vi "DCAM_show_preview_update_camera.vi"() -> ()   [LabVIEW 2015]
panel:
  out "S Horiz Width":i32
  in  "Horizontal Width":i32 min=4 max=2048 step=4
  out "Image Preview":u16[][](graph) caption="Image"
  out "S Start Trig Mode":dbl
  out "S Binning":dbl
  in  "Start Trigger Mode":u32(ring)=1 items=["Internal"=1, "External Edge"=2, "External Level"=4, "Software"=32, "Fast Repetition"=64, "TDI"=128, "Trigger Start"=512, "Sync Readout"=1024]
  in  "Binning":u16(ring) items=["1x1"=1, "2x2"=2, "4x4"=4]
  out "S Vert Offset":i32
  out "S Horiz Offset":i32
  in  "Vertical Offset":i32 min=0 max=0 step=4
  in  "Horizontal Offset":i32 min=0 max=0 step=4
  in  "Scan Mode":dbl min=1.0 max=2.0 step=1.0
  out "S Scan Mode":dbl min=1.0 max=2.0 step=1.0
  in  "Exposure":dbl min=0.0010036691729323308 max=10.000004210526315 step=1e-08
  out "S Exposure":dbl
  out "S Vert Width":i32
  in  "Vertical Width":i32 min=4 max=2048 step=4
  out "error out":errorcluster
  out "DCAM Ver.":string
  out "Library Ver.":string
  out "Firmware":string
  out "Camera ID":string
  out "Model":string
  out "Timeseries Base Filename":string
  out "Timeseries Save Path":path
  in  "Start Button":bool
  out "Image":u16[][](graph)
  in  "Stop":bool
  out "Frames Recorded":i32
  in  "Frames":i32=100
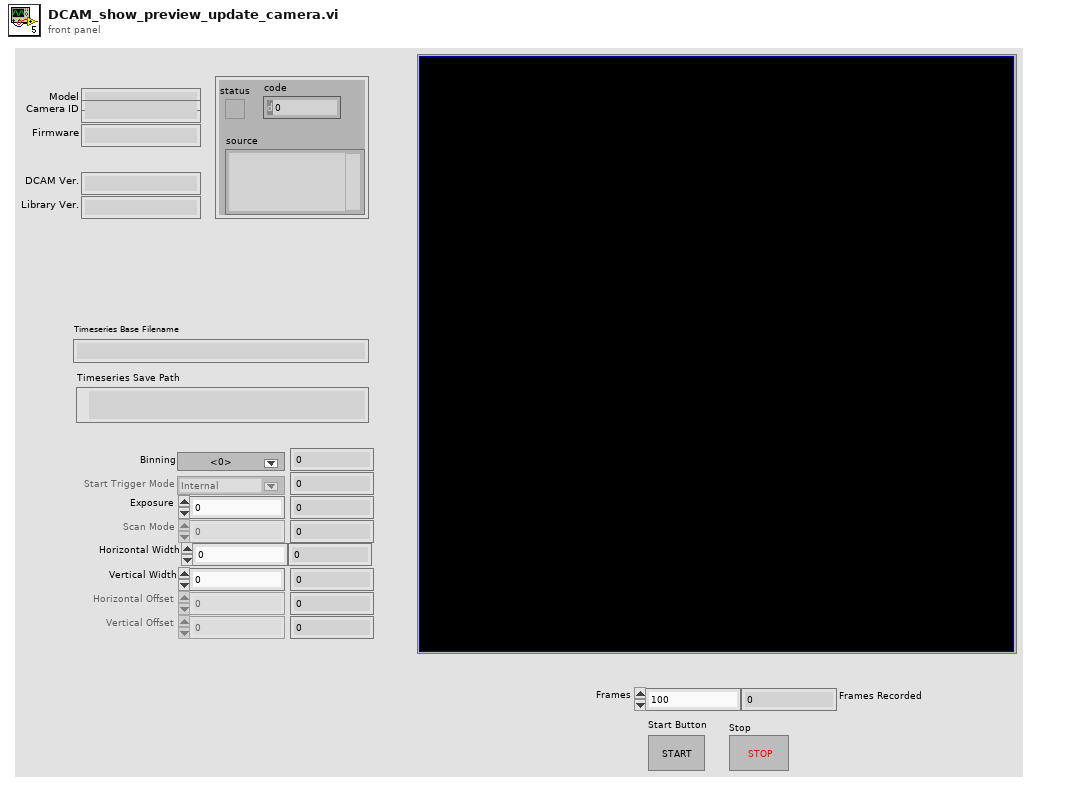
[diagram p1: front panel]
types:
  T1 = cluster{"Capture Library":string, "DCAM-API":string}
  T2 = cluster{"Model":string, "Camera ID":string, "Firmware":string}
  T3 = cluster{"Value":i32, "Minimum":i32, "Maximum":i32, "Increment":i32}
  T4 = cluster{"height":u32, "width":u32, "datatype":u32}
  T5 = cluster{"Horizontal Offset":i32, "Vertical Offset":i32, "Horizontal Width":i32, "Vertical Width":i32}
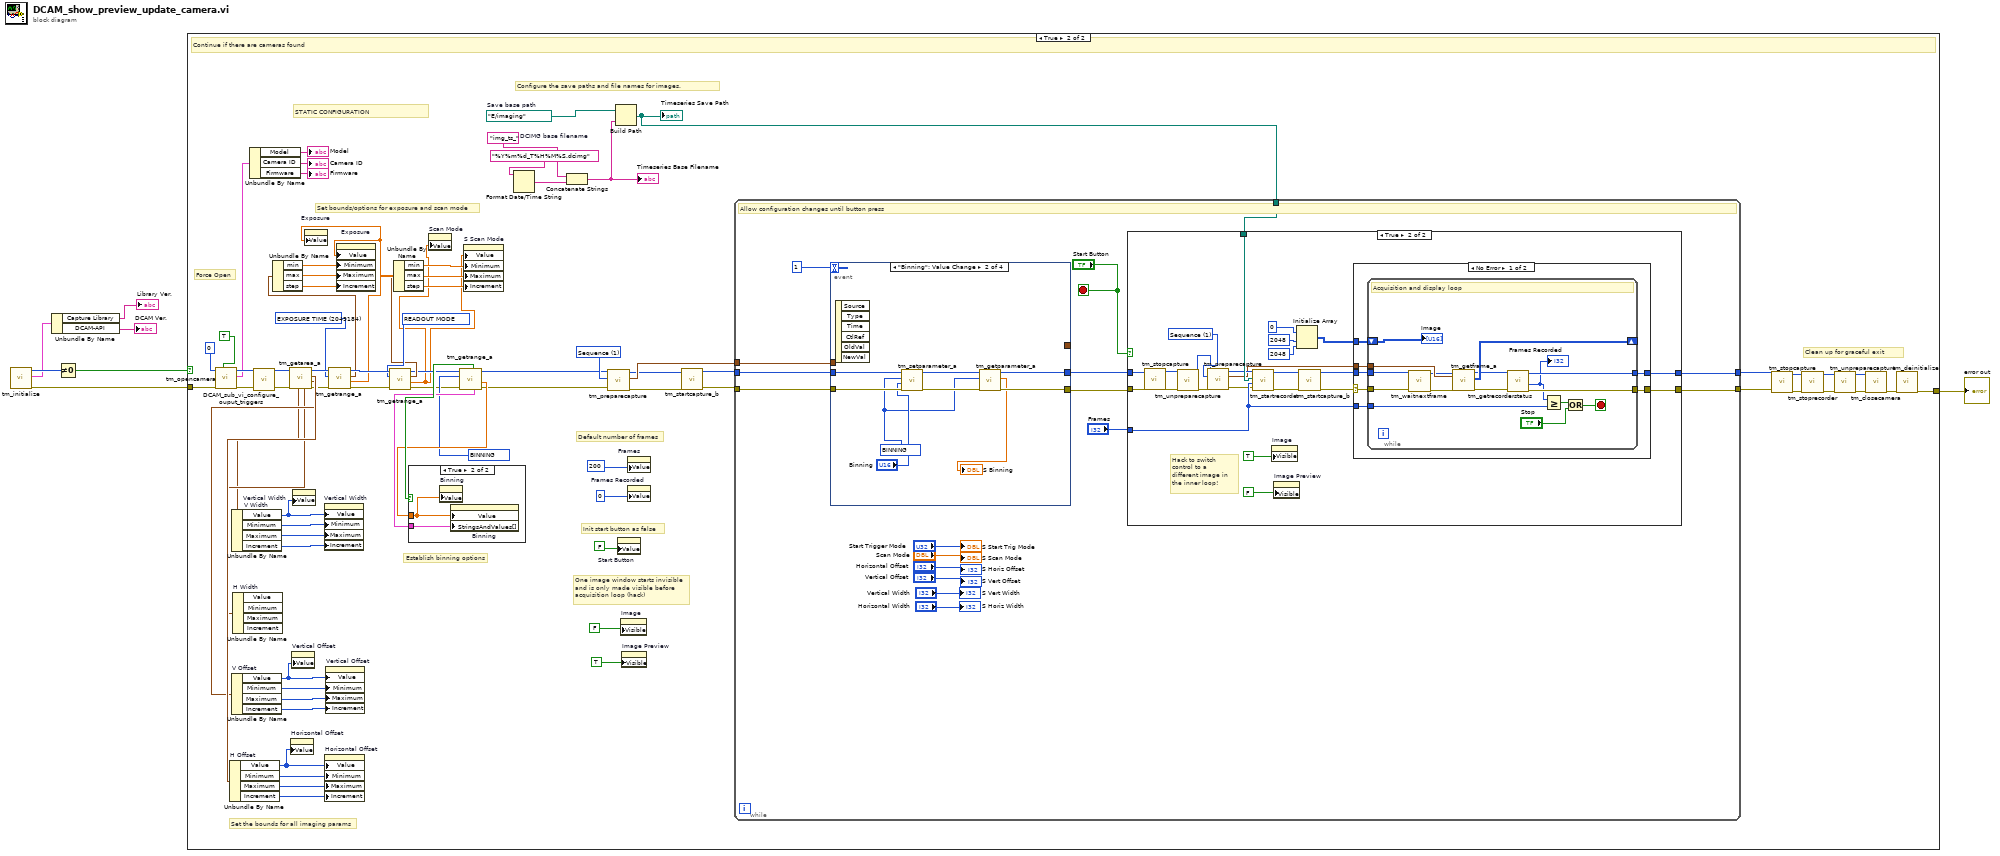
[diagram p0: block diagram]
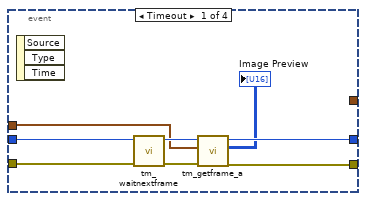
[diagram p4: hidden frame]
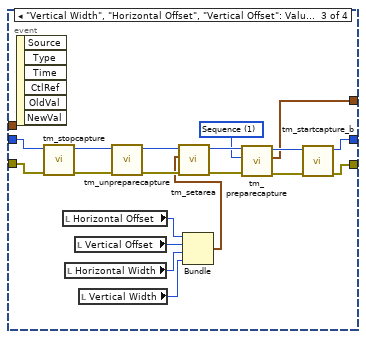
[diagram p5: hidden frame]
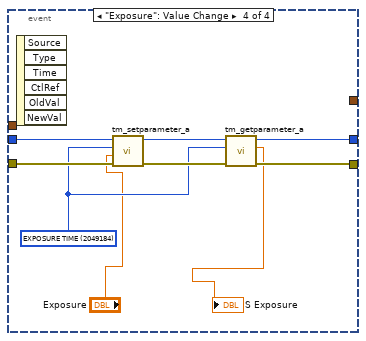
[diagram p6: hidden frame]
diagram:
  n1 = call <userlib>:"tm_initialize.vi"() -> ("error out"=w2:errorcluster, "Version Info"=w5:T1, "Number Of Cameras"=w7:u32)  [unwired: 8 in, 1 out]
  n2 = Unbundle By Name(w5) -> ("Capture Library"=→"Library Ver.":string, "DCAM-API"=→"DCAM Ver.":string)
  n3 = Not Equal To 0?(x=w7) -> (x != 0?=w6:bool)
  n4 = case shown="True" w6 {
    tunnel: w2 -> [w8 w85]
    tunnel: [w8 w74] -> w1
    frame False {
    }
    frame True {
      w22 = u32 4215968 items=["BINNING"=4215968, "BITS PER CHANNEL"=4342976, "ACTIVE VIEW INDEX"=4343136, "CCD MODE"=4212384, "SENSOR MODE"=4212128, "READOUT MODE"=4211872, "EXPOSURE TIME"=2049184, "CONTRAST GAIN"=3163312, "CONTRAST OFFSET"=3163328, "LIGHT MODE"=2114720, "SENSITIVITY"=2114992, "WHITE BALANCE"=3163568, "PHOTON IMAGING MODE"=2115200, "HIGH DYNAMIC RANGE MODE"=3163360, "TRIGGER SOURCE"=1066144, "TRIGGER ACTIVE"=1066160, "TRIGGER MODE"=1066400, "TRIGGER POLARITY"=1066416, "TRIGGER GLOBAL EXPOSURE"=2049680, "FIRST TRIGGER BEHAVIOR"=2049696, "TRIGGER TIMES"=1066448, "OUTPUT TRIGGER POLARITY"=1852592, "OUTPUT TRIGGER DELAY"=1852624, "OUTPUT TRIGGER PERIOD"=1852640, "TEMPERATURE"=2115232, "TEMPERATURE TARGET"=2115264, "SENSOR COOLER FAN"=2115296, "MECHANICAL SHUTTER"=2115488, "BACK FOCUS POSITION"=8422304, "FRAMEBUNDLE MODE"=4346784, "FRAMEBUNDLE NUMBER"=4346800, "LINEBUNDLE HEIGHT"=4212192, "TRIGGER CONNECTOR"=1066432, "IMAGE PIXEL TYPE"=4343296, "OUTPUT TRIGGER KIND"=1852656, "READOUT DIRECTION"=4211904, "CHANNEL SYNC"=1852352] ("Parameter")
      w28 = u32 4211872 items=["BINNING"=4215968, "BITS PER CHANNEL"=4342976, "ACTIVE VIEW INDEX"=4343136, "CCD MODE"=4212384, "SENSOR MODE"=4212128, "READOUT MODE"=4211872, "EXPOSURE TIME"=2049184, "CONTRAST GAIN"=3163312, "CONTRAST OFFSET"=3163328, "LIGHT MODE"=2114720, "SENSITIVITY"=2114992, "WHITE BALANCE"=3163568, "PHOTON IMAGING MODE"=2115200, "HIGH DYNAMIC RANGE MODE"=3163360, "TRIGGER SOURCE"=1066144, "TRIGGER ACTIVE"=1066160, "TRIGGER MODE"=1066400, "TRIGGER POLARITY"=1066416, "TRIGGER GLOBAL EXPOSURE"=2049680, "FIRST TRIGGER BEHAVIOR"=2049696, "TRIGGER TIMES"=1066448, "OUTPUT TRIGGER POLARITY"=1852592, "OUTPUT TRIGGER DELAY"=1852624, "OUTPUT TRIGGER PERIOD"=1852640, "TEMPERATURE"=2115232, "TEMPERATURE TARGET"=2115264, "SENSOR COOLER FAN"=2115296, "MECHANICAL SHUTTER"=2115488, "BACK FOCUS POSITION"=8422304, "FRAMEBUNDLE MODE"=4346784, "FRAMEBUNDLE NUMBER"=4346800, "LINEBUNDLE HEIGHT"=4212192, "TRIGGER CONNECTOR"=1066432, "IMAGE PIXEL TYPE"=4343296, "OUTPUT TRIGGER KIND"=1852656, "READOUT DIRECTION"=4211904, "CHANNEL SYNC"=1852352] ("Parameter")
      w33 = u32 2049184 items=["BINNING"=4215968, "BITS PER CHANNEL"=4342976, "ACTIVE VIEW INDEX"=4343136, "CCD MODE"=4212384, "SENSOR MODE"=4212128, "READOUT MODE"=4211872, "EXPOSURE TIME"=2049184, "CONTRAST GAIN"=3163312, "CONTRAST OFFSET"=3163328, "LIGHT MODE"=2114720, "SENSITIVITY"=2114992, "WHITE BALANCE"=3163568, "PHOTON IMAGING MODE"=2115200, "HIGH DYNAMIC RANGE MODE"=3163360, "TRIGGER SOURCE"=1066144, "TRIGGER ACTIVE"=1066160, "TRIGGER MODE"=1066400, "TRIGGER POLARITY"=1066416, "TRIGGER GLOBAL EXPOSURE"=2049680, "FIRST TRIGGER BEHAVIOR"=2049696, "TRIGGER TIMES"=1066448, "OUTPUT TRIGGER POLARITY"=1852592, "OUTPUT TRIGGER DELAY"=1852624, "OUTPUT TRIGGER PERIOD"=1852640, "TEMPERATURE"=2115232, "TEMPERATURE TARGET"=2115264, "SENSOR COOLER FAN"=2115296, "MECHANICAL SHUTTER"=2115488, "BACK FOCUS POSITION"=8422304, "FRAMEBUNDLE MODE"=4346784, "FRAMEBUNDLE NUMBER"=4346800, "LINEBUNDLE HEIGHT"=4212192, "TRIGGER CONNECTOR"=1066432, "IMAGE PIXEL TYPE"=4343296, "OUTPUT TRIGGER KIND"=1852656, "READOUT DIRECTION"=4211904, "CHANNEL SYNC"=1852352] ("Parameter")
      w73 = 1 items=["Snap", "Sequence"] ("Capture mode")
      w62 = "img_ts_"  # DCIMG base filename
      w65 = path "E:/imaging"  # Save base path
      # "One image window starts invisible and is only made visible before acquisition loop (hack)"
      # "Force Open"
      # "STATIC CONFIGURATION"
      # "Set bounds/options for exposure and scan mode"
      # "Establish binning options"
      # "Set the bounds for all imaging params"
      # "Init start button as false"
      # "Clean up for graceful exit"
      # "Default number of frames"
      # "Configure the save paths and file names for images."
      # "Continue if there are cameras found"
      n5 = call <userlib>:"tm_opencamera.vi"("Force Open"=TRUE, "error in (no error)"=w85, "Camera Index"=0) -> ("error out"=w82:errorcluster, "Camera Details"=w78:T2, "Handle out"=w83:u32)  [unwired: 6 in]
      n6 = Unbundle By Name(w78) -> ("Model"=→"Model":string, "Camera ID"=→"Camera ID":string, "Firmware"=→"Firmware":string)
      n7 = call "DCAM_sub_vi_configure_ouput_triggers.vi"("error in (no error)"=w82, "Handle in"=w83) -> ("error out"=w47:errorcluster, "Handle out"=w48:u32)  [unwired: 2 in]
      n8 = call <userlib>:"tm_getarea_a.vi"("error in (no error)"=w47, "Handle in"=w48) -> ("error out"=w40:errorcluster, "V Offset"=w43:T3, "H Offset"=w46:T3, "Handle out"=w45:u32, "H Width"=w42:T3, "V Width"=w41:T3)  [unwired: 4 in]
      n9 = Unbundle By Name "H Offset"(w46) -> ("Value"=w38:i32, "Minimum"=w51:i32, "Maximum"=w50:i32, "Increment"=w49:i32)
      n10 = Unbundle By Name "V Width"(w41) -> ("Value"=w36:i32, "Minimum"=w57:i32, "Maximum"=w56:i32, "Increment"=w55:i32)
      n11 = Unbundle By Name "V Offset"(w43) -> ("Value"=w37:i32, "Minimum"=w54:i32, "Maximum"=w53:i32, "Increment"=w52:i32)
      n12 = Unbundle By Name "H Width"(w42) -> ()  [unwired: 4 out]
      n13 = property on="Horizontal Offset" class="DigNum (strict)"("Value"=w38) -> ()  [unwired: 2 in, 2 out]
      n14 = property on="Vertical Offset" class="DigNum (strict)"("Value"=w37) -> ()  [unwired: 2 in, 2 out]
      n15 = property on="Vertical Width" class="DigNum (strict)"("Value"=w36) -> ()  [unwired: 2 in, 2 out]
      n16 = property on="Vertical Width" class="DigNum (strict)"("Value"=w36, "Minimum"=w57, "Maximum"=w56, "Increment"=w55) -> ()  [unwired: 2 in, 2 out]
      n17 = property on="Horizontal Offset" class="DigNum (strict)"("Value"=w38, "Minimum"=w51, "Maximum"=w50, "Increment"=w49) -> ()  [unwired: 2 in, 2 out]
      n18 = property on="Vertical Offset" class="DigNum (strict)"("Value"=w37, "Minimum"=w54, "Maximum"=w53, "Increment"=w52) -> ()  [unwired: 2 in, 2 out]
      n19 = call <userlib>:"tm_getrange_a.vi"("error in (no error)"=w40, "Parameter"=w33, "Handle in"=w45) -> ("error out"=w39:errorcluster, "default"=w17:dbl, "Range"=w32:cluster{"min":dbl, "max":dbl, "step":dbl}, "Handle out"=w44:u32)  [unwired: 2 in, 3 out]
      n20 = Unbundle By Name(w32) -> ("min"=w31:dbl, "max"=w34:dbl, "step"=w35:dbl)
      n21 = property on="Exposure" class="DigNum (strict)"("Value"=w17) -> ()  [unwired: 2 in, 2 out]
      n22 = property on="Exposure" class="DigNum (strict)"("Value"=w17, "Minimum"=w31, "Maximum"=w34, "Increment"=w35) -> ()  [unwired: 2 in, 2 out]
      n23 = call <userlib>:"tm_getrange_a.vi"("error in (no error)"=w39, "Parameter"=w28, "Handle in"=w44) -> ("error out"=w20:errorcluster, "default"=w16:dbl, "Range"=w27:cluster{"min":dbl, "max":dbl, "step":dbl}, "Handle out"=w21:u32)  [unwired: 2 in, 3 out]
      n24 = Unbundle By Name(w27) -> ("min"=w26:dbl, "max"=w29:dbl, "step"=w30:dbl)
      n25 = property on="Scan Mode" class="DigNum (strict)"("Value"=w16) -> ()  [unwired: 2 in, 2 out]
      n26 = call <userlib>:"tm_getrange_a.vi"("error in (no error)"=w20, "Parameter"=w22, "Handle in"=w21) -> ("error out"=w18:errorcluster, "default"=w24:dbl, "Handle out"=w19:u32, "Value Names"=w23:cluster{"Name":string, "Value":dbl}[], "Writable"=w25:bool)  [unwired: 2 in, 2 out]
      n27 = case shown="True" w25 {
        tunnel: w23 -> [_ w88]
        tunnel: w24 -> [_ w87]
        frame False {
        }
        frame True {
          n28 = property on="Binning" class="Ring (strict)"("Value"=w87) -> ()  [unwired: 2 in, 2 out]
          n29 = property on="Binning" class="Ring (strict)"("Value"=w87, "StringsAndValues[]"=w88) -> ()  [unwired: 2 in, 2 out]
        }
      }
      n30 = property on="S Scan Mode" class="DigNum (strict)"("Value"=w16, "Minimum"=w26, "Maximum"=w29, "Increment"=w30) -> ()  [unwired: 2 in, 2 out]
      n31 = Format Date/Time String(time format string (%c)="%Y%m%d_T%H%M%S.dcimg" ("name or relative path")) -> (date/time string=w63:string)  [unwired: 2 in]
      n32 = Concatenate Strings(w62, w63) -> (w60:string)
      "Timeseries Base Filename" <- w60
      n33 = call <userlib>:"tm_preparecapture.vi"("error in (no error)"=w18, "Capture mode"=w73, "Handle in"=w19) -> ("error out"=w10:errorcluster, "Buffer Info"=w14:T4, "Handle out"=w13:u32)  [unwired: 5 in, 1 out]
      n34 = Build Path(base path=w65, name or relative path=w60) -> (appended path=w61:path)
      "Timeseries Save Path" <- w61
      n35 = property on="Start Button" class="Bool (strict)"("Value"=FALSE) -> ()  [unwired: 2 in, 2 out]
      n36 = property on="Image" class="IntGraph (strict)"("Visible"=FALSE) -> ()  [unwired: 2 in, 2 out]
      n37 = property on="Image Preview" class="IntGraph (strict)"("Visible"=TRUE) -> ()  [unwired: 2 in, 2 out]
      n38 = property on="Frames" class="DigNum (strict)"("Value"=200) -> ()  [unwired: 2 in, 2 out]
      n39 = property on="Frames Recorded" class="DigNum (strict)"("Value"=0) -> ()  [unwired: 2 in, 2 out]
      n40 = call <userlib>:"tm_startcapture_b.vi"("error in (no error)"=w10, "Handle in"=w13) -> ("error out"=w11:errorcluster, "Handle out"=w12:u32)  [unwired: 8 in]
      n41 = while {
        tunnel: w14 -> [w96]
        tunnel: w61 -> [w103]
        tunnel: w11 -> [w95]
        tunnel: [w104] -> w70
        tunnel: w12 -> [w94]
        tunnel: [w105] -> w71
        stop <- "Start Button" stop-if-true
        # "Allow configuration changes until button press"
        n42 = event shown="[1] \"Binning\": Value Change" {
          selector: _ -> [_ _ _ _]
          dyn-events: _ -> [_ _ _ _]
          timeout: 1 -> [_ _ _ _]
          tunnel: w96 -> [w111 _ _ _]
          tunnel: w95 -> [w106 w122 w136 w150]
          tunnel: w94 -> [w107 w121 w131 w149]
          tunnel: [w110 w116 w130 w145] -> w92
          tunnel: [w109 w118 w137 w147] -> w93
          tunnel: [_ _ w129 _] -> _
          event Timeout {
            n43 = event-data() -> ()  [unwired: 1 in, 3 out]
            n44 = call <userlib>:"tm_waitnextframe.vi"("error in (no error)"=w106, "Handle in"=w107) -> ("error out"=w113:errorcluster, "Handle out"=w112:u32)  [unwired: 6 in, 2 out]
            n45 = call <userlib>:"tm_getframe_a.vi"("error in (no error)"=w113, "Buffer Info"=w111, "Handle in"=w112) -> ("error out"=w109:errorcluster, "Data 16"=→"Image Preview":u16[][], "Handle out"=w110:u32)  [unwired: 4 in, 2 out]
          }
          event "Binning": Value Change {
            w114 = u32 4215968 items=["SUBARRAY HPOS"=4220064, "SUBARRAY VPOS"=4220096, "SUBARRAY VSIZE"=4220112, "SUBARRAY HSIZE"=4220080, "BINNING"=4215968, "BITS PER CHANNEL"=4342976, "ACTIVE VIEW INDEX"=4343136, "CCD MODE"=4212384, "SENSOR MODE"=4212128, "READOUT MODE"=4211872, "EXPOSURE TIME"=2049184, "CONTRAST GAIN"=3163312, "CONTRAST OFFSET"=3163328, "LIGHT MODE"=2114720, "SENSITIVITY"=2114992, "WHITE BALANCE"=3163568, "PHOTON IMAGING MODE"=2115200, "HIGH DYNAMIC RANGE MODE"=3163360, "TRIGGER SOURCE"=1066144, "TRIGGER ACTIVE"=1066160, "TRIGGER MODE"=1066400, "TRIGGER POLARITY"=1066416, "TRIGGER GLOBAL EXPOSURE"=2049680, "FIRST TRIGGER BEHAVIOR"=2049696, "TRIGGER TIMES"=1066448, "OUTPUT TRIGGER POLARITY"=1852592, "OUTPUT TRIGGER DELAY"=1852624, "OUTPUT TRIGGER PERIOD"=1852640, "TEMPERATURE"=2115232, "TEMPERATURE TARGET"=2115264, "SENSOR COOLER FAN"=2115296, "MECHANICAL SHUTTER"=2115488, "BACK FOCUS POSITION"=8422304, "FRAMEBUNDLE MODE"=4346784, "FRAMEBUNDLE NUMBER"=4346800, "LINEBUNDLE HEIGHT"=4212192, "TRIGGER CONNECTOR"=1066432, "IMAGE PIXEL TYPE"=4343296, "OUTPUT TRIGGER KIND"=1852656, "READOUT DIRECTION"=4211904, "CHANNEL SYNC"=1852352] ("Parameter")
            n46 = event-data() -> ()  [unwired: 1 in, 6 out]
            n47 = call <userlib>:"tm_setparameter_a.vi"("error in (no error)"=w122, "Value in"="Binning", "Parameter"=w114, "Handle in"=w121) -> ("error out"=w119:errorcluster, "Handle out"=w117:u32)  [unwired: 6 in]
            n48 = call <userlib>:"tm_getparameter_a.vi"("error in (no error)"=w119, "Parameter"=w114, "Handle in"=w117) -> ("error out"=w118:errorcluster, "Value out"=→"S Binning":dbl, "Handle out"=w116:u32)  [unwired: 6 in]
          }
          event "Vertical Width", "Horizontal Offset", "Vertical Offset": Value Change {
            w123 = 1 items=["Snap", "Sequence"] ("Capture mode")
            n49 = event-data() -> ()  [unwired: 1 in, 6 out]
            n50 = call <userlib>:"tm_stopcapture.vi"("error in (no error)"=w136, "Handle in"=w131) -> ("error out"=w141:errorcluster, "Handle out"=w132:u32)  [unwired: 8 in]
            n51 = local read "Horizontal Offset"() -> (w125:i32)
            n52 = local read "Horizontal Width"() -> (w126:i32)
            n53 = local read "Vertical Offset"() -> (w124:i32)
            n54 = local read "Vertical Width"() -> (w127:i32)
            n55 = call <userlib>:"tm_unpreparecapture.vi"("error in (no error)"=w141, "Handle in"=w132) -> ("error out"=w140:errorcluster, "Handle out"=w135:u32)  [unwired: 8 in]
            n56 = Bundle("Horizontal Offset"=w125, "Vertical Offset"=w124, "Horizontal Width"=w126, "Vertical Width"=w127) -> (w128:T5)  [unwired: 1 in]
            n57 = call <userlib>:"tm_setarea.vi"("error in (no error)"=w140, "Sub Region"=w128, "Handle in"=w135) -> ("error out"=w139:errorcluster, "Handle out"=w134:u32)  [unwired: 7 in]
            n58 = call <userlib>:"tm_preparecapture.vi"("error in (no error)"=w139, "Capture mode"=w123, "Handle in"=w134) -> ("error out"=w138:errorcluster, "Buffer Info"=w129:T4, "Handle out"=w133:u32)  [unwired: 5 in, 1 out]
            n59 = call <userlib>:"tm_startcapture_b.vi"("error in (no error)"=w138, "Handle in"=w133) -> ("error out"=w137:errorcluster, "Handle out"=w130:u32)  [unwired: 8 in]
          }
          event "Exposure": Value Change {
            w144 = u32 2049184 items=["BINNING"=4215968, "BITS PER CHANNEL"=4342976, "ACTIVE VIEW INDEX"=4343136, "CCD MODE"=4212384, "SENSOR MODE"=4212128, "READOUT MODE"=4211872, "EXPOSURE TIME"=2049184, "CONTRAST GAIN"=3163312, "CONTRAST OFFSET"=3163328, "LIGHT MODE"=2114720, "SENSITIVITY"=2114992, "WHITE BALANCE"=3163568, "PHOTON IMAGING MODE"=2115200, "HIGH DYNAMIC RANGE MODE"=3163360, "TRIGGER SOURCE"=1066144, "TRIGGER ACTIVE"=1066160, "TRIGGER MODE"=1066400, "TRIGGER POLARITY"=1066416, "TRIGGER GLOBAL EXPOSURE"=2049680, "FIRST TRIGGER BEHAVIOR"=2049696, "TRIGGER TIMES"=1066448, "OUTPUT TRIGGER POLARITY"=1852592, "OUTPUT TRIGGER DELAY"=1852624, "OUTPUT TRIGGER PERIOD"=1852640, "TEMPERATURE"=2115232, "TEMPERATURE TARGET"=2115264, "SENSOR COOLER FAN"=2115296, "MECHANICAL SHUTTER"=2115488, "BACK FOCUS POSITION"=8422304, "FRAMEBUNDLE MODE"=4346784, "FRAMEBUNDLE NUMBER"=4346800, "LINEBUNDLE HEIGHT"=4212192, "TRIGGER CONNECTOR"=1066432, "IMAGE PIXEL TYPE"=4343296, "OUTPUT TRIGGER KIND"=1852656, "READOUT DIRECTION"=4211904, "CHANNEL SYNC"=1852352] ("Parameter")
            n60 = event-data() -> ()  [unwired: 1 in, 6 out]
            n61 = call <userlib>:"tm_setparameter_a.vi"("error in (no error)"=w150, "Value in"="Exposure", "Parameter"=w144, "Handle in"=w149) -> ("error out"=w148:errorcluster, "Handle out"=w146:u32)  [unwired: 6 in]
            n62 = call <userlib>:"tm_getparameter_a.vi"("error in (no error)"=w148, "Parameter"=w144, "Handle in"=w146) -> ("error out"=w147:errorcluster, "Value out"=→"S Exposure":dbl, "Handle out"=w145:u32)  [unwired: 6 in]
          }
        }
        n63 = case shown="True" "Start Button" {
          tunnel: w92 -> [w152 w157]
          tunnel: w93 -> [w151 w156]
          tunnel: [w152 w169] -> w105
          tunnel: [w151 w168] -> w104
          tunnel: "Frames" -> [_ w167]
          tunnel: w103 -> [_ w165]
          frame False {
          }
          frame True {
            w164 = 1 items=["Snap", "Sequence"] ("Capture mode")
            # "Hack to switch control to a different image in the inner loop!"
            n64 = call <userlib>:"tm_stopcapture.vi"("error in (no error)"=w156, "Handle in"=w157) -> ("error out"=w158:errorcluster, "Handle out"=w155:u32)  [unwired: 8 in]
            n65 = call <userlib>:"tm_unpreparecapture.vi"("error in (no error)"=w158, "Handle in"=w155) -> ("error out"=w153:errorcluster, "Handle out"=w154:u32)  [unwired: 8 in]
            n66 = call <userlib>:"tm_preparecapture.vi"("error in (no error)"=w153, "Capture mode"=w164, "Handle in"=w154) -> ("error out"=w161:errorcluster, "Buffer Info"=w162:T4, "Handle out"=w163:u32)  [unwired: 5 in, 1 out]
            n67 = call <userlib>:"tm_startrecorder.vi"("error in (no error)"=w161, "frames"=w167, "File"=w165, "Handle in"=w163) -> ("error out"=w171:errorcluster, "Handle out"=w170:u32)  [unwired: 6 in]
            n68 = property on="Image" class="IntGraph (strict)"("Visible"=TRUE) -> ()  [unwired: 2 in, 2 out]
            n69 = property on="Image Preview" class="IntGraph (strict)"("Visible"=FALSE) -> ()  [unwired: 2 in, 2 out]
            n70 = Initialize Array(u16 0 ("element"), 2048 ("dimension size"), 2048 ("dimension size")) -> (w172:u16[][])
            n71 = call <userlib>:"tm_startcapture_b.vi"("error in (no error)"=w171, "Handle in"=w170) -> ("error out"=w166:errorcluster, "Handle out"=w176:u32)  [unwired: 8 in]
            n72 = case shown="No Error" w166 {
              selector: w166 -> [w177 w201]
              tunnel: w162 -> [w183 _]
              tunnel: w176 -> [w182 w200]
              tunnel: w172 -> [w181 _]
              tunnel: [w180 w200] -> w169
              tunnel: [w179 w201] -> w168
              tunnel: w167 -> [w178 _]
              frame No Error {
                n73 = while {
                  tunnel: w183 -> [w199]
                  tunnel: w182 -> [w198]
                  tunnel: w177 -> [w195]
                  shift-right: [w194] -> _
                  shift-left: w181 -> [w184]
                  tunnel: [w191] -> w180
                  tunnel: [w190] -> w179
                  tunnel: w178 -> [w185]
                  stop <- w188 stop-if-true
                  # "Acquisition and display loop"
                  n74 = call <userlib>:"tm_waitnextframe.vi"("error in (no error)"=w195, "Handle in"=w198) -> ("error out"=w196:errorcluster, "Handle out"=w197:u32)  [unwired: 6 in, 2 out]
                  n75 = call <userlib>:"tm_getframe_a.vi"("error in (no error)"=w196, "Buffer Info"=w199, "Handle in"=w197) -> ("error out"=w193:errorcluster, "Data 16"=w194:u16[][], "Handle out"=w192:u32)  [unwired: 4 in, 2 out]
                  n76 = call <userlib>:"tm_getrecorderstatus.vi"("error in (no error)"=w193, "Handle"=w192) -> ("error out"=w190:errorcluster, "Count"=w186:i32, "Handle"=w191:u32)  [unwired: 6 in, 1 out]
                  "Frames Recorded" <- w186
                  n77 = Greater Or Equal?(x=w186, y=w185) -> (x >= y?=w187:bool)
                  n78 = Or(x=w187, y="Stop") -> (x .or. y?=w188:bool)
                  "Image" <- w184
                }
              }
              frame Error {
              }
            }
          }
        }
        "S Scan Mode" <- "Scan Mode"
        "S Vert Offset" <- "Vertical Offset"
        "S Horiz Offset" <- "Horizontal Offset"
        "S Start Trig Mode" <- "Start Trigger Mode"
        "S Vert Width" <- "Vertical Width"
        "S Horiz Width" <- "Horizontal Width"
      }
      n79 = call <userlib>:"tm_stopcapture.vi"("error in (no error)"=w70, "Handle in"=w71) -> ("error out"=w66:errorcluster, "Handle out"=w67:u32)  [unwired: 8 in]
      n80 = call <userlib>:"tm_stoprecorder.vi"("error in (no error)"=w66, "Handle in"=w67) -> ("error out"=w68:errorcluster, "Handle out"=w69:u32)  [unwired: 8 in]
      n81 = call <userlib>:"tm_unpreparecapture.vi"("error in (no error)"=w68, "Handle in"=w69) -> ("error out"=w77:errorcluster, "Handle out"=w76:u32)  [unwired: 8 in]
      n82 = call <userlib>:"tm_closecamera.vi"("error in (no error)"=w77, "Handle in"=w76) -> ("error out"=w75:errorcluster)  [unwired: 9 in]
      n83 = call <userlib>:"tm_deinitialize.vi"("error in (no error)"=w75) -> ("error out"=w74:errorcluster)  [unwired: 10 in]
    }
  }
  "error out" <- w1
